vi "Read csv.vi"(8 "error in (no error)":errorcluster) -> (0 "error out":errorcluster, 3 "Zone Setup":cluster{"Zone Selector":string, "Timing":dbl}[](array[cluster]))   [LabVIEW 2015]
uses:
  <vilib>/Utility/file.llb/Read Delimited Spreadsheet (string).vi
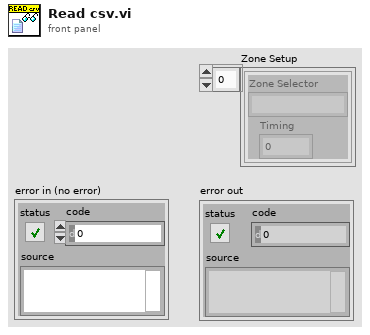
[diagram p1: front panel]
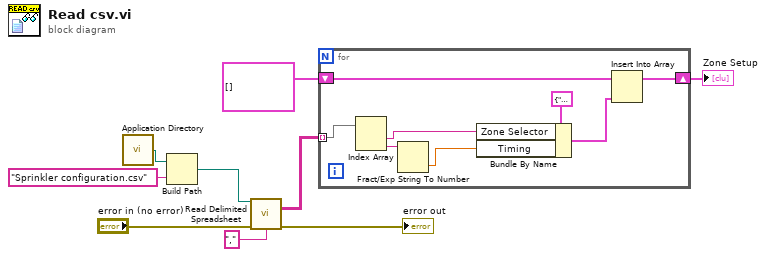
[diagram p0: block diagram]
diagram:
  n1 = call <vilib>:"Application Directory.vi"() -> ("Application Directory"=w1:path)
  n2 = Build Path(base path=w1, name or relative path="Sprinkler configuration.csv") -> (appended path=w3:path)
  n3 = call-poly <vilib>:"Read Delimited Spreadsheet.vi"("file path (dialog if empty)"=w3, "error in (no error)"="error in (no error)", "delimiter (\\t)"="," ("delimiter (\\t)")) -> ("all rows"=w5:string[][], "error out"=→"error out":errorcluster)  [unwired: 7 in, 4 out]
  n4 = for {
    tunnel: w5 -> [w17] mode=indexing
    shift-right: [w14] -> w9
    shift-left: cluster{"Zone Selector":string, "Timing":dbl}[] [] ("Zone Setup Array 2") -> [w15]
    n5 = Index Array(array=w17) -> (element #1=w11:string, element #2=w16:string)  [unwired: 2 in]
    n6 = Fract/Exp String To Number(string=w16) -> (number=w12:dbl)  [unwired: 3 in, 1 out]
    n7 = Bundle By Name(cluster=cluster{"Zone Selector":string, "Timing":dbl} {"Zone Selector"="", "Timing"=0.0} ("new element/subarray"), "Zone Selector"=w11, "Timing"=w12) -> (w10:cluster{"Zone Selector":string, "Timing":dbl})
    n8 = Insert Into Array(array=w15, new element=w10) -> (w14:cluster{"Zone Selector":string, "Timing":dbl}[])  [unwired: 1 in]
  }
  "Zone Setup" <- w9
